vi "PhaseToSLM.vi"() -> ()   [LabVIEW 2019]
uses:
  PCIe16LabVIEWSDK/Interface.dll
  <vilib>/vision/NI_Vision_Development_Module.lvlib
panel:
  out "Phase Image":u16[][](array[numeric])
  out "SLM":bool
  in  "Start SLM":bool
  out "Update SLM":bool
  out "PCIe16SDK Path":string
  out "Board ID":i32
  out "# of Boards":i32
  in  "Phase Image Path":path
  out "Phase Image":T1(plugin-control)
  out "Init.":bool
  in  "Stop":bool
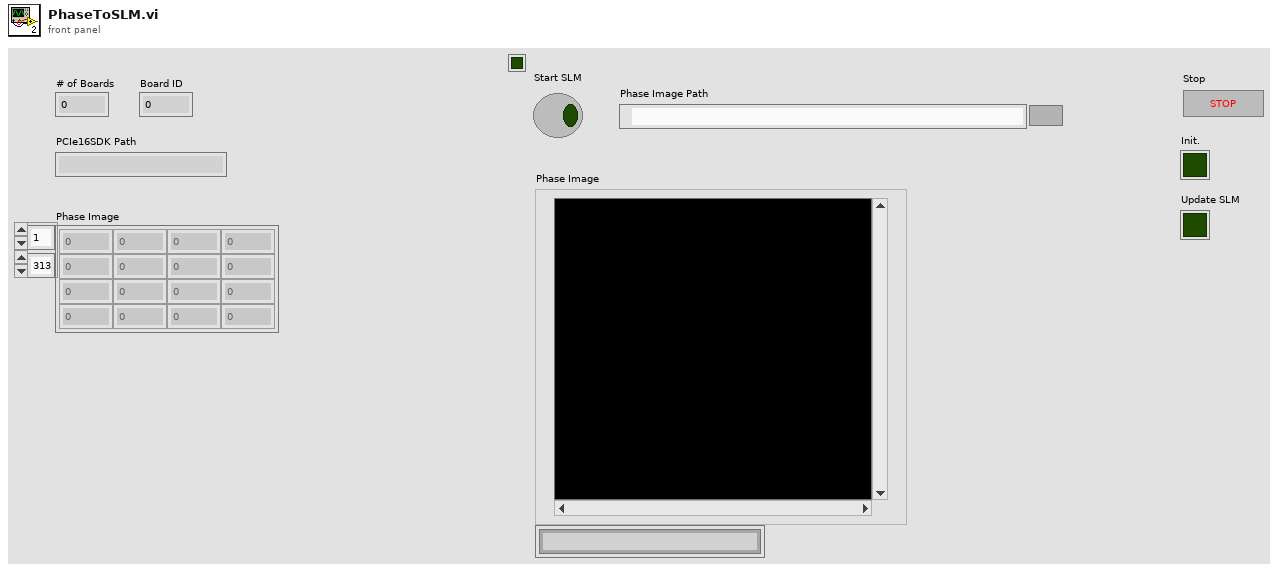
[diagram p1: front panel]
types:
  T1 = typedef "IMAQ Image.ctl" = refnum<image>
  T2 = typedef "Image Type" = u32
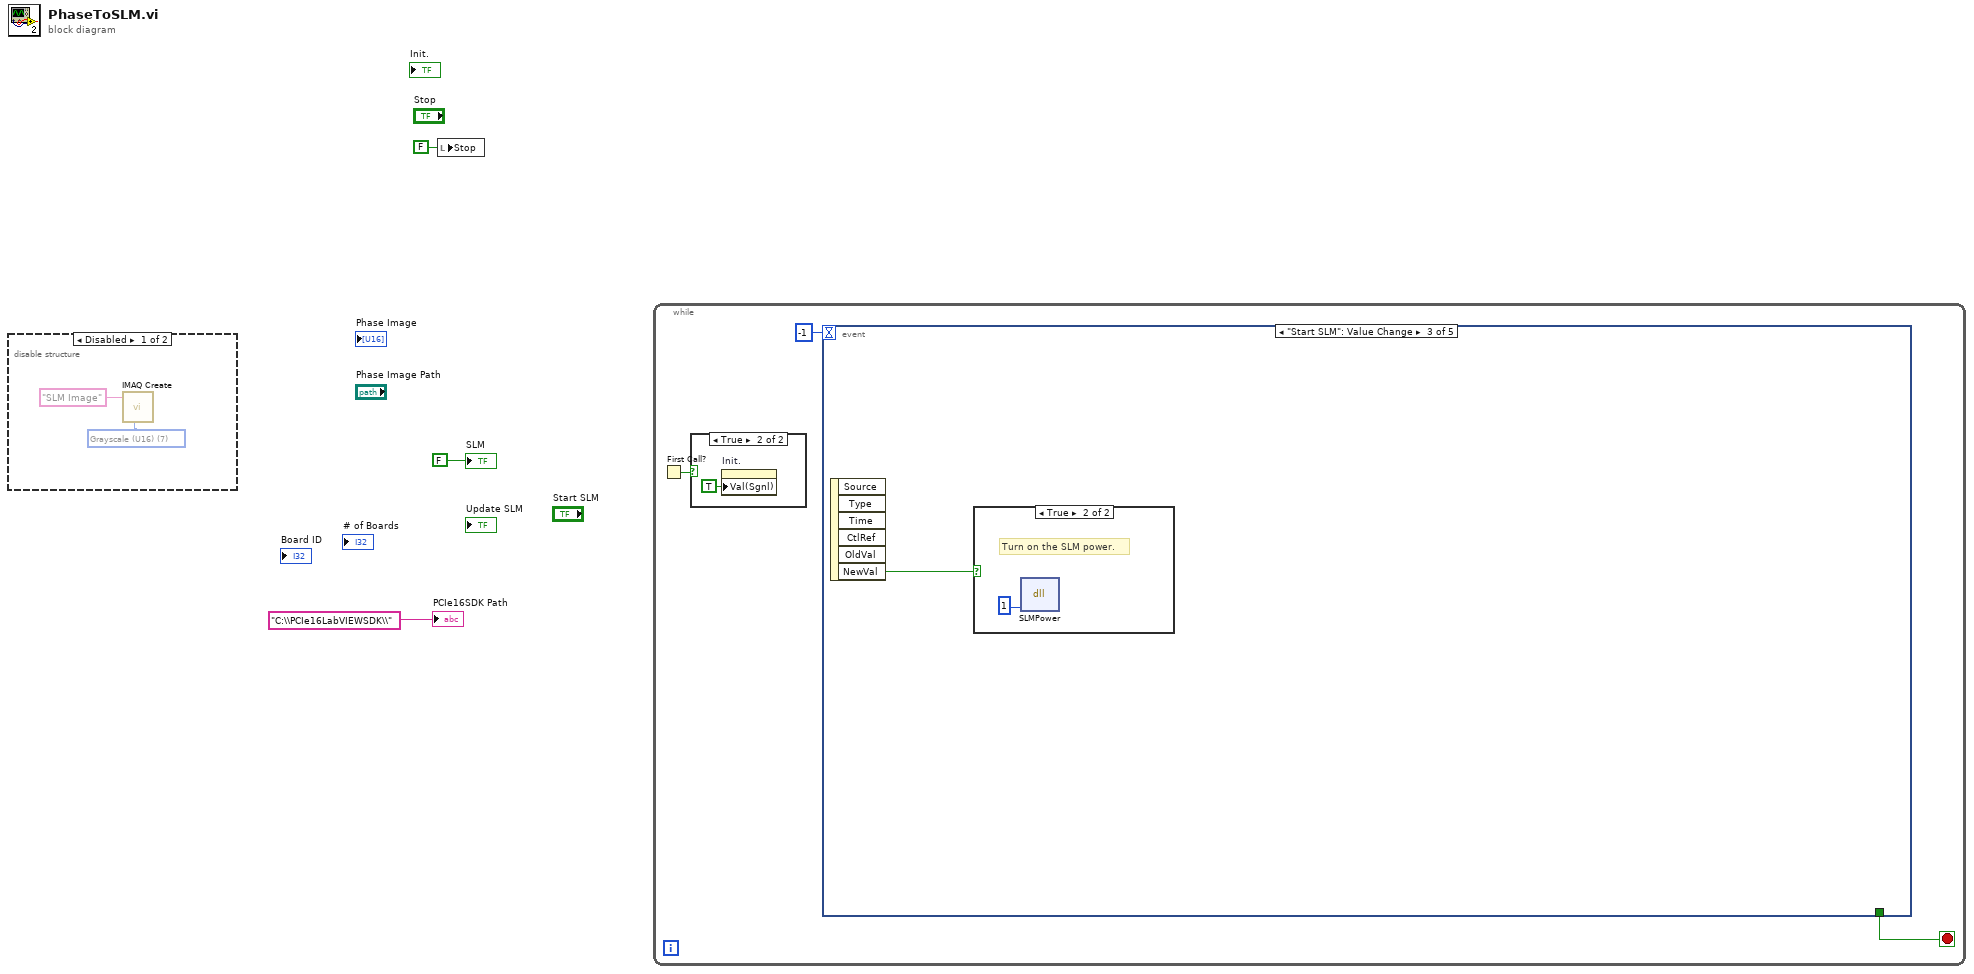
[diagram p0: block diagram]
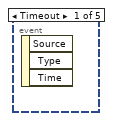
[diagram p4: hidden frame]
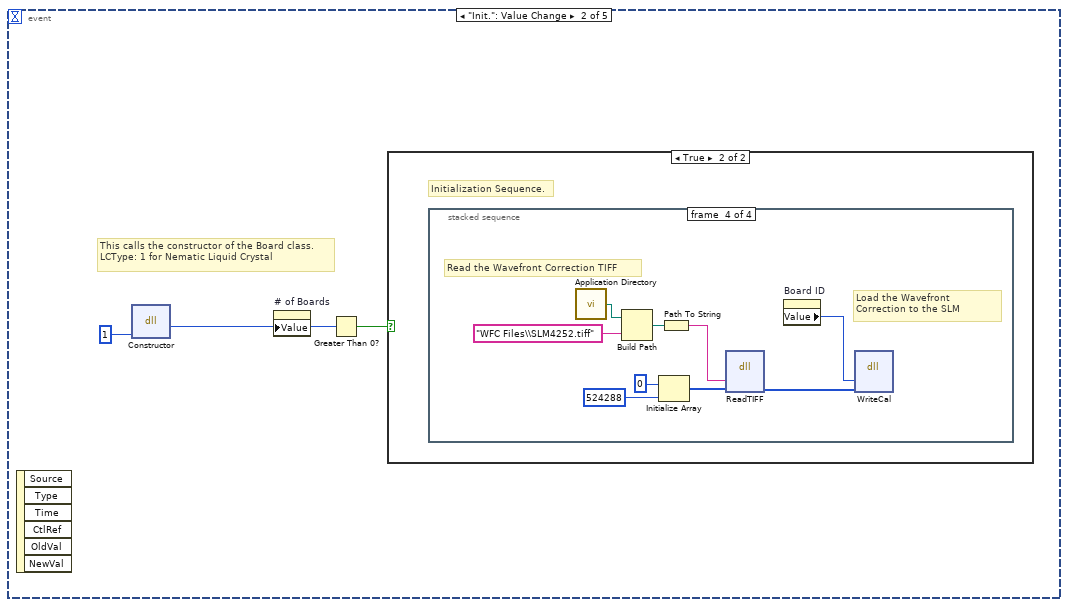
[diagram p5: hidden frame]
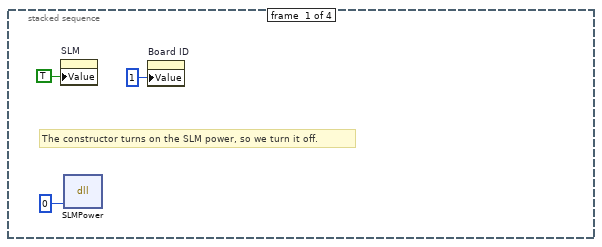
[diagram p7: hidden frame]
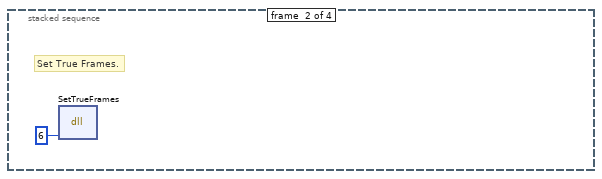
[diagram p8: hidden frame]
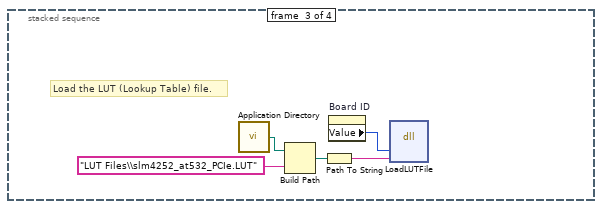
[diagram p9: hidden frame]
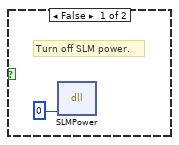
[diagram p10: hidden frame]
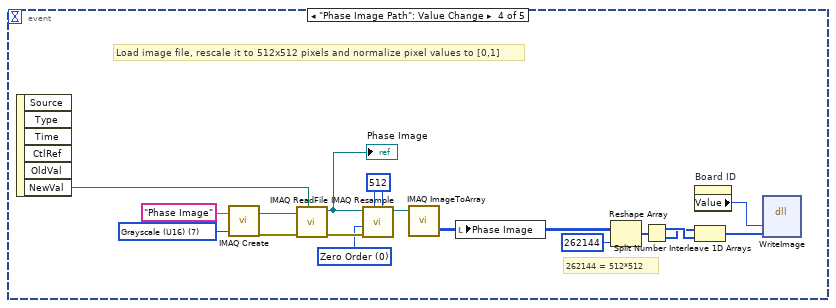
[diagram p11: hidden frame]
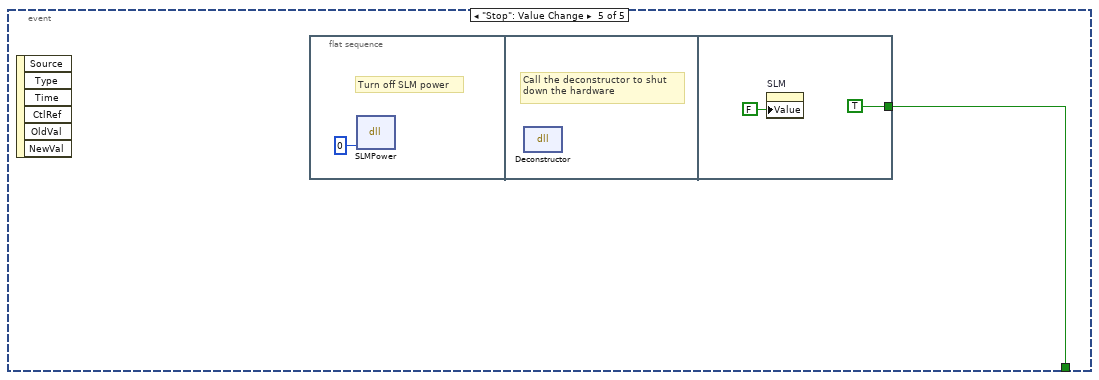
[diagram p12: hidden frame]
diagram:
  n1 = disable-structure shown="Disabled" {
    frame Disabled {
      w4 = T2 7 items=["Grayscale (U8)", "Grayscale (I16)", "Grayscale (SGL)", "Complex (CSG)", "RGB (U32)", "HSL (U32)", "RGB (U64)", "Grayscale (U16)"] ("Image Type")
      n2 = call "IMAQ Create"("Image Name"="SLM Image", "Image Type"=w4) -> ()  [unwired: 3 in, 2 out]
    }
    frame Enabled {
    }
  }
  n3 = local write "Stop"(FALSE ("Stop")) -> ()
  n4 = while {
    stop <- w7 stop-if-true
    n5 = First Call?() -> (First Call?: T/F=w6:bool)
    n6 = case shown="True" w6 {
      frame False {
      }
      frame True {
        n7 = property on="Init." class="Bool (strict)"("Val(Sgnl)"=TRUE ("Value (Signaling)")) -> ()  [unwired: 2 in, 2 out]
      }
    }
    n8 = event shown="[2] \"Start SLM\": Value Change" {
      selector: _ -> [_ _ _ _ _]
      dyn-events: _ -> [_ _ _ _ _]
      timeout: -1 -> [_ _ _ _ _]
      tunnel: [_ _ _ _ w51] -> w7
      event Timeout {
        n9 = event-data() -> ()  [unwired: 1 in, 3 out]
      }
      event "Init.": Value Change {
        # "This calls the constructor of the Board class. LCType: 1 for Nematic Liquid Crystal"
        n10 = event-data() -> ()  [unwired: 1 in, 6 out]
        n11 = dll-call lib="C:/PCIe16LabVIEWSDK/Interface.dll" fn="Constructor"("LCType"=u8 1) -> ("return type"=w10:i32)  [unwired: 4 in, 2 out]
        n12 = property on="# of Boards" class="DigNum (strict)"("Value"=w10) -> ()  [unwired: 2 in, 2 out]
        n13 = Greater Than 0?(x=w10) -> (x > 0?=w12:bool)
        n14 = case shown="True" w12 {
          frame False {
          }
          frame True {
            # "Initialization Sequence."
            n15 = stacked-sequence {
              frame #0 {
                # "The constructor turns on the SLM power, so we turn it off."
                n16 = property on="SLM" class="Bool (strict)"("Value"=TRUE ("SLM")) -> ()  [unwired: 2 in, 2 out]
                n17 = dll-call lib="C:/PCIe16LabVIEWSDK/Interface.dll" fn="SLMPower"("PowerState"=0) -> ()  [unwired: 5 in, 2 out]
                n18 = property on="Board ID" class="DigNum (strict)"("Value"=1 ("Board Number")) -> ()  [unwired: 2 in, 2 out]
              }
              frame #1 {
                # "Set True Frames."
                n19 = dll-call lib="C:/PCIe16LabVIEWSDK/Interface.dll" fn="SetTrueFrames"("TrueFrames"=6) -> ()  [unwired: 5 in, 2 out]
              }
              frame #2 {
                # "Load the LUT (Lookup Table) file."
                n20 = call <vilib>:"Application Directory.vi"() -> ("Application Directory"=w19:path)
                n21 = Build Path(base path=w19, name or relative path="LUT Files\\slm4252_at532_PCIe.LUT") -> (appended path=w20:path)
                n22 = Path To String(path=w20) -> (string=w17:string)
                n23 = property on="Board ID" class="DigNum (strict)"() -> ("Value"=w21:i32)  [unwired: 2 in, 2 out]
                n24 = dll-call lib="C:/PCIe16LabVIEWSDK/Interface.dll" fn="LoadLUTFile"("board"=w21, "LUTPath"=w17) -> ()  [unwired: 6 in, 2 out]
              }
              frame #3 {
                # "Read the Wavefront Correction TIFF"
                # "Load the Wavefront Correction to the SLM"
                n25 = call <vilib>:"Application Directory.vi"() -> ("Application Directory"=w27:path)
                n26 = Build Path(base path=w27, name or relative path="WFC Files\\SLM4252.tiff") -> (appended path=w28:path)
                n27 = Initialize Array(u8 0, 524288) -> (w22:u8[])
                n28 = Path To String(path=w28) -> (string=w25:string)
                n29 = dll-call lib="C:/PCIe16LabVIEWSDK/Interface.dll" fn="ReadTIFF"("TiffPath"=w25, "Image"=w22) -> ("Image"=w30:u8[])  [unwired: 5 in, 2 out]
                n30 = property on="Board ID" class="DigNum (strict)"() -> ("Value"=w29:i32)  [unwired: 2 in, 2 out]
                n31 = dll-call lib="C:/PCIe16LabVIEWSDK/Interface.dll" fn="WriteCal"("board"=w29, "Image"=w30) -> ()  [unwired: 6 in, 2 out]
              }
            }
          }
        }
      }
      event "Start SLM": Value Change {
        n32 = event-data() -> ("NewVal"=w31:bool)  [unwired: 1 in, 5 out]
        n33 = case shown="True" w31 {
          frame False {
            # "Turn off SLM power."
            n34 = dll-call lib="C:/PCIe16LabVIEWSDK/Interface.dll" fn="SLMPower"("PowerState"=0) -> ()  [unwired: 5 in, 2 out]
          }
          frame True {
            # "Turn on the SLM power."
            n35 = dll-call lib="C:/PCIe16LabVIEWSDK/Interface.dll" fn="SLMPower"("PowerState"=1) -> ()  [unwired: 5 in, 2 out]
          }
        }
      }
      event "Phase Image Path": Value Change {
        w43 = T2 7 items=["Grayscale (U8)", "Grayscale (I16)", "Grayscale (SGL)", "Complex (CSG)", "RGB (U32)", "HSL (U32)", "RGB (U64)", "Grayscale (U16)"] ("Image Type")
        w46 = 512
        w45 = u32 0 items=["Zero Order", "Bi-Linear", "Quadratic", "Cubic Spline"] ("Interpolation Type")
        # "262144 = 512*512"
        # "Load image file, rescale it to 512x512 pixels and normalize pixel values to [0,1]"
        n36 = event-data() -> ("NewVal"=w42:path)  [unwired: 1 in, 5 out]
        n37 = call "IMAQ Create"("Image Name"="Phase Image", "Image Type"=w43) -> ("New Image"=w47:T1, "error out"=w48:errorcluster)  [unwired: 3 in]
        n38 = call "IMAQ ReadFile"("File Path"=w42, "error in (no error)"=w48, "Image"=w47) -> ("error out"=w49:errorcluster, "Image Out"=w41:T1)  [unwired: 4 in, 3 out]
        "Phase Image" <- w41
        n39 = call "IMAQ Resample"("X Resolution"=w46, "Y Resolution"=w46, "error in (no error)"=w49, "Interpolation Type"=w45, "Image Src"=w41) -> ("Image Dst Out"=w50:T1)  [unwired: 5 in, 1 out]
        n40 = call "IMAQ ImageToArray"("Image"=w50) -> ("Image Pixels (U16)"=w34:u16[][])  [unwired: 3 in, 4 out]
        n41 = local write "Phase Image"(w34) -> ()
        n42 = Reshape Array(w34, 262144 ("dimension size")) -> (w37:u16[])
        n43 = Split Number(x=w37) -> (hi(x)=w40:u8[], lo(x)=w39:u8[])
        n44 = property on="Board ID" class="DigNum (strict)"() -> ("Value"=w36:i32)  [unwired: 2 in, 2 out]
        n45 = Interleave 1D Arrays(w39, w40) -> (w38:u8[])
        n46 = dll-call lib="C:/PCIe16LabVIEWSDK/Interface.dll" fn="WriteImage"("board"=w36, "Image"=w38) -> ()  [unwired: 6 in, 2 out]
      }
      event "Stop": Value Change {
        n47 = event-data() -> ()  [unwired: 1 in, 6 out]
        n48 = flat-sequence {
          tunnel: [TRUE] -> w51
          frame #0 {
            # "Turn off SLM power"
            n49 = dll-call lib="C:/PCIe16LabVIEWSDK/Interface.dll" fn="SLMPower"("PowerState"=0) -> ()  [unwired: 5 in, 2 out]
          }
          frame #1 {
            # "Call the deconstructor to shut \ndown the hardware"
            n50 = dll-call lib="C:/PCIe16LabVIEWSDK/Interface.dll" fn="Deconstructor"() -> ()  [unwired: 4 in, 2 out]
          }
          frame #2 {
            n51 = property on="SLM" class="Bool (strict)"("Value"=FALSE ("SLM")) -> ()  [unwired: 2 in, 2 out]
          }
        }
      }
    }
  }
  "PCIe16SDK Path" <- "C:\\PCIe16LabVIEWSDK\\"
  "SLM" <- FALSE
